vi "ResetChannelVI.vi"(0 "Angelsample":dbl[](array[numeric]), 1 "Angel":bool[](array[boolean]), 2 "dt":dbl, 5 "Torquesample":dbl[](array[numeric]), 7 "Torque":bool[](array[boolean]), 9 "ResetAngel":dbl[](array[numeric]), 11 "ResetTorque":dbl[](array[numeric]), 12 "ChannelSetArray":T1[](array[typedef]) {"Enable" items=["不使能", "使能"]; "Wave" items=["0指令", "正弦波", "方波", "三角波", "常值", "波形数据", "白噪声", "正弦扫频", "梯度加载", "VMIC"]; "ChannelType" items=["标准波形跟踪"=1, "扫频测试"=2, "消除多余力"=3, "梯度加载"=4, "载荷谱跟踪"=5, "模拟输入跟踪"=9]; "ChannelStatus" items=["通道关", "位置通道", "加载通道"]}, 13 "ControlPara":dbl[][](array[numeric])) -> (4 "OutPut":dbl[](array[numeric]), 6 "resetAngel 2":dbl[](array[numeric]), 10 "ResetTorque 2":dbl[](array[numeric]), 15 "Commandout":dbl[](array[numeric]))   [LabVIEW 2011]
uses:
  ChannelCommand.ctl
  Control 1.ctl
  WaveType.ctl
  MoterEnable.ctl
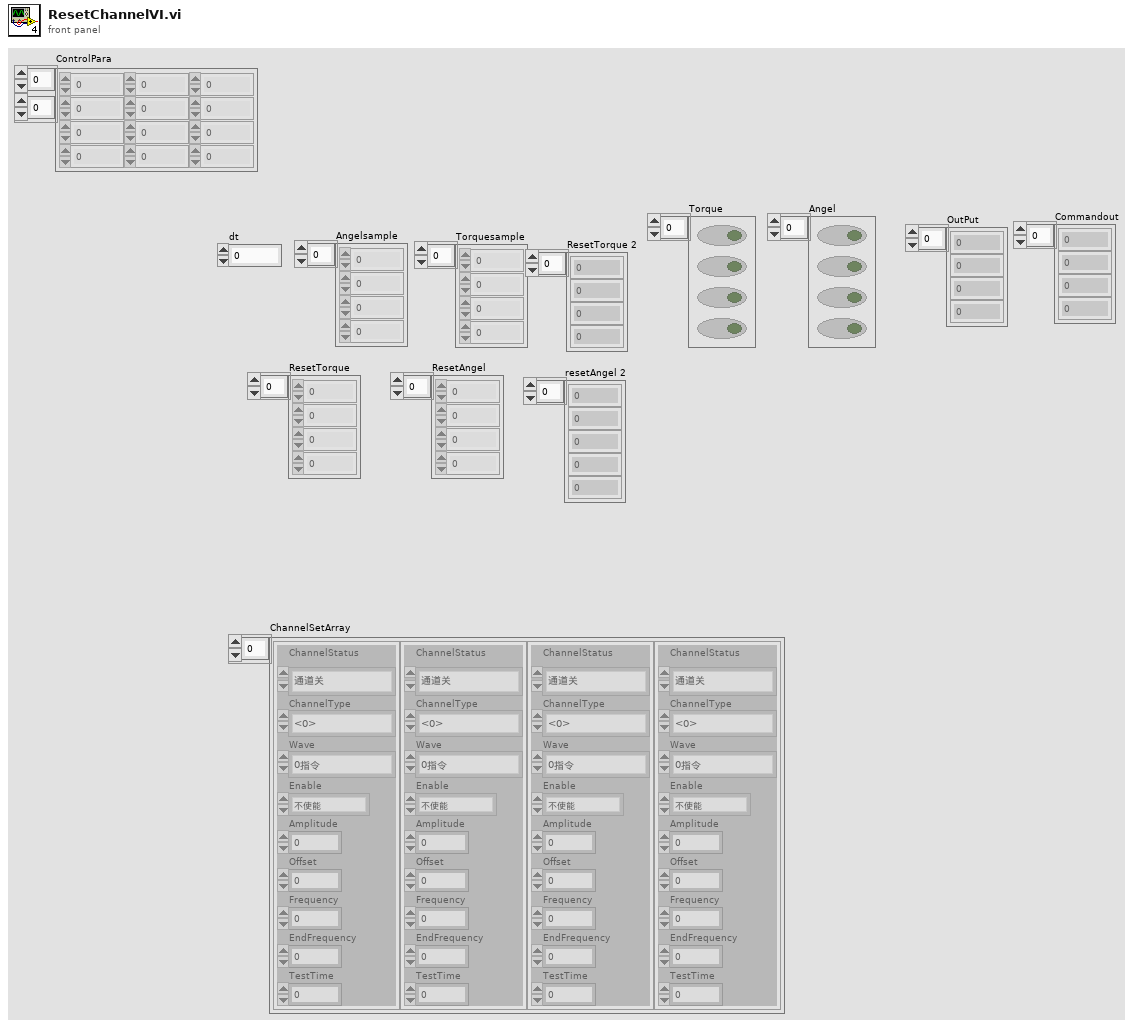
[diagram p1: front panel]
types:
  T1 = typedef "ChannelCommand.ctl" = cluster{"ChannelStatus":T2, "ChannelType":i32, "Wave":T3, "Enable":T4, "Amplitude":dbl, "Offset":dbl, "Frequency":dbl, "EndFrequency":dbl, "TestTime":dbl}
  T2 = typedef "Control 1.ctl" = i32
  T3 = typedef "WaveType.ctl" = i32
  T4 = typedef "MoterEnable.ctl" = u16
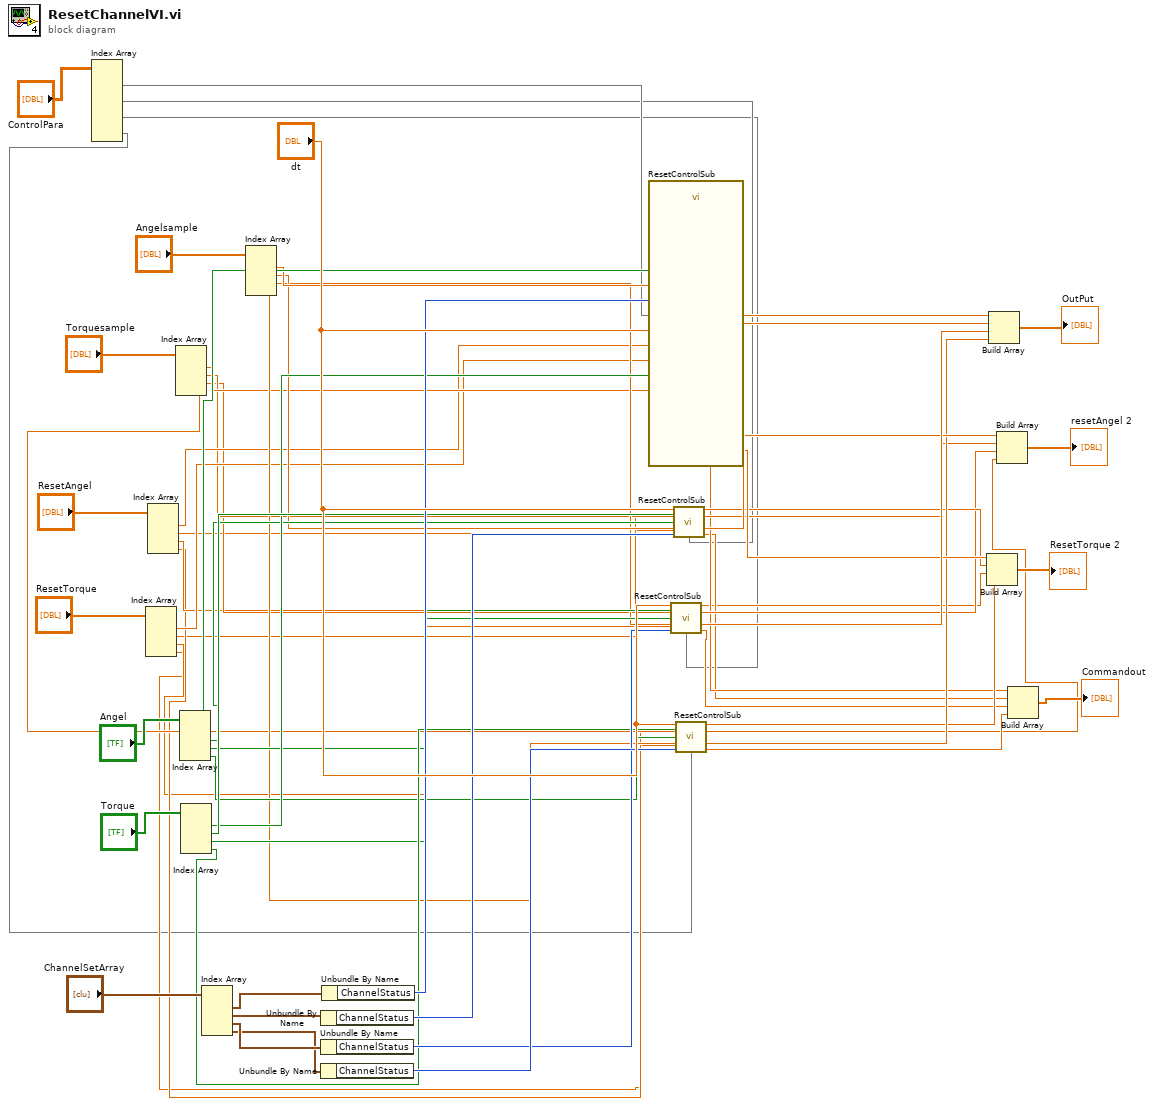
[diagram p0: block diagram]
diagram:
  n1 = Index Array(array="ControlPara") -> (element #1=w4:dbl[], element #2=w3:dbl[], element #3=w2:dbl[], element #4=w1:dbl[])  [unwired: 8 in]
  n2 = Index Array(array="ResetTorque") -> (element #1=w32:dbl, element #2=w25:dbl, element #3=w24:dbl, element #4=w23:dbl)  [unwired: 4 in]
  n3 = Index Array(array="ResetAngel") -> (element #1=w33:dbl, element #2=w28:dbl, element #3=w27:dbl, element #4=w26:dbl)  [unwired: 4 in]
  n4 = Index Array(array="Torquesample") -> (element #1=w34:dbl, element #2=w31:dbl, element #3=w30:dbl, element #4=w29:dbl)  [unwired: 4 in]
  n5 = Index Array(array="Angel") -> (element #1=w39:bool, element #2=w40:bool, element #3=w41:bool, element #4=w42:bool)  [unwired: 4 in]
  n6 = Index Array(array="Torque") -> (element #1=w43:bool, element #2=w44:bool, element #3=w45:bool, element #4=w46:bool)  [unwired: 4 in]
  n7 = Index Array(array="ChannelSetArray") -> (element #1=w57:T1, element #2=w56:T1, element #3=w55:T1, element #4=w54:T1)  [unwired: 4 in]
  n8 = Index Array(array="Angelsample") -> (element #1=w38:dbl, element #2=w37:dbl, element #3=w36:dbl, element #4=w35:dbl)  [unwired: 4 in]
  n9 = Unbundle By Name(w56) -> ("ChannelStatus"=w50:T2)
  n10 = Unbundle By Name(w55) -> ("ChannelStatus"=w51:T2)
  n11 = Unbundle By Name(w54) -> ("ChannelStatus"=w52:T2)
  n12 = Unbundle By Name(w57) -> ("ChannelStatus"=w49:T2)
  n13 = call "ResetControlSub.vi"("dt"="dt", "Torque"=w43, "ResetAngle"=w33, "TorqueSample0"=w34, "Angel"=w39, "AngleSample0"=w38, "ChannelStatus"=w49, "ResetTorque"=w32, "ControlPara"=w4) -> ("ResetTorque 2"=w18:dbl, "ResetAngle 2"=w19:dbl, "ControlOutput"=w22:dbl, "Commandout"=w11:dbl)  [unwired: 3 in]
  n14 = call "ResetControlSub.vi"("dt"="dt", "Torque"=w45, "ResetAngle"=w27, "TorqueSample0"=w30, "Angel"=w41, "AngleSample0"=w36, "ChannelStatus"=w51, "ResetTorque"=w24, "ControlPara"=w2) -> ("ResetTorque 2"=w7:dbl, "ResetAngle 2"=w14:dbl, "ControlOutput"=w20:dbl, "Commandout"=w9:dbl)  [unwired: 3 in]
  n15 = call "ResetControlSub.vi"("dt"="dt", "Torque"=w44, "ResetAngle"=w28, "TorqueSample0"=w31, "Angel"=w40, "AngleSample0"=w37, "ChannelStatus"=w50, "ResetTorque"=w25, "ControlPara"=w3) -> ("ResetTorque 2"=w15:dbl, "ResetAngle 2"=w16:dbl, "ControlOutput"=w21:dbl, "Commandout"=w10:dbl)  [unwired: 3 in]
  n16 = call "ResetControlSub.vi"("dt"="dt", "Torque"=w46, "ResetAngle"=w26, "TorqueSample0"=w29, "Angel"=w42, "AngleSample0"=w35, "ChannelStatus"=w52, "ResetTorque"=w23, "ControlPara"=w1) -> ("ResetTorque 2"=w13:dbl, "ResetAngle 2"=w6:dbl, "ControlOutput"=w17:dbl, "Commandout"=w8:dbl)  [unwired: 3 in]
  n17 = Build Array(w18, w15, w7, w13) -> (→"ResetTorque 2":dbl[])
  n18 = Build Array(w22, w21, w20, w17) -> (→"OutPut":dbl[])
  n19 = Build Array(w19, w16, w14, w6) -> (→"resetAngel 2":dbl[])
  n20 = Build Array(w11, w10, w9, w8) -> (→"Commandout":dbl[])
